vi "Win Host - New Selections.vi"(8 "error in (no error)":errorcluster, 10 "New Item Names":string[](array[string]), 11 "ListBox in":refnum<vi>) -> (0 "error out":errorcluster, 3 "ListBox out":refnum<vi>)   [LabVIEW 2024]
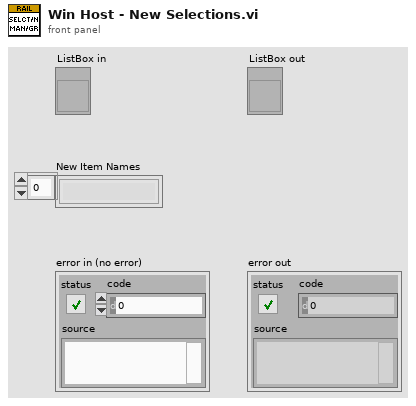
[diagram p1: front panel]
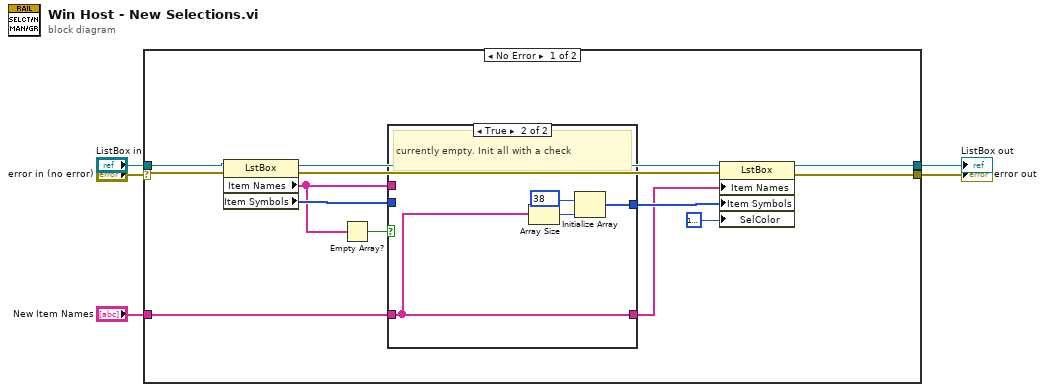
[diagram p0: block diagram]
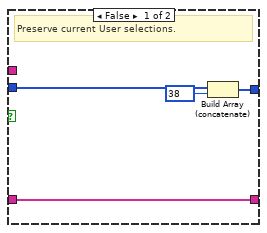
[diagram p2: hidden frame]
diagram:
  n1 = case shown="No Error" "error in (no error)" {
    selector: "error in (no error)" -> [w12 w27]
    tunnel: "New Item Names" -> [w17 _]
    tunnel: [w16 w28] -> w4
    tunnel: [w15 w27] -> w3
    tunnel: "ListBox in" -> [w13 w28]
    frame No Error {
      n2 = property class="LstBox"(reference=w13, error in=w12) -> (reference out=w10:refnum<vi>, error out=w11:errorcluster, "Item Names"=w7:string[], "Item Symbols"=w8:i32[])
      n3 = Empty Array?(array=w7) -> (empty?=w9:bool)
      n4 = case shown="True" w9 {
        tunnel: w17 -> [w19 w23]
        tunnel: [w21 w26] -> w14
        tunnel: w8 -> [w20 _]
        tunnel: w7 -> [_ _]
        tunnel: [w19 w23] -> w6
        frame False {
          # "Preserve current User selections."
          n5 = Build Array (concatenate)(w20, 38) -> (w21:i32[])
        }
        frame True {
          # "currently empty. Init all with a check"
          n6 = Array Size(array=w23) -> (size(s)=w24:i32)
          n7 = Initialize Array(38, w24) -> (w26:i32[])
        }
      }
      n8 = property class="LstBox"(reference=w10, error in=w11, "Item Names"=w6, "Item Symbols"=w14, "SelColor"=u32 16777225) -> (reference out=w16:refnum<vi>, error out=w15:errorcluster)
    }
    frame Error {
    }
  }
  "ListBox out" <- w4
  "error out" <- w3
